vi "Firmware.vi"() -> ()   [LabVIEW 2025]
doc: "VI para instalar el Firmware en las ESP32 \nCon la opcion de subir el firmware en modo Online u Offline"
panel:
  in  "Stop Button":bool
  out "Progreso":u8(slide) scale=0.0..100.0
  out "Compilado":bool
  out "Subido":bool
  in  "Upload Firmware":bool
  out "Lista de COMs":string[](array[string])
  out "error out":errorcluster
  in  "Selector":string(combo)
  # "Instalador de Firmware de Labview ESP32"
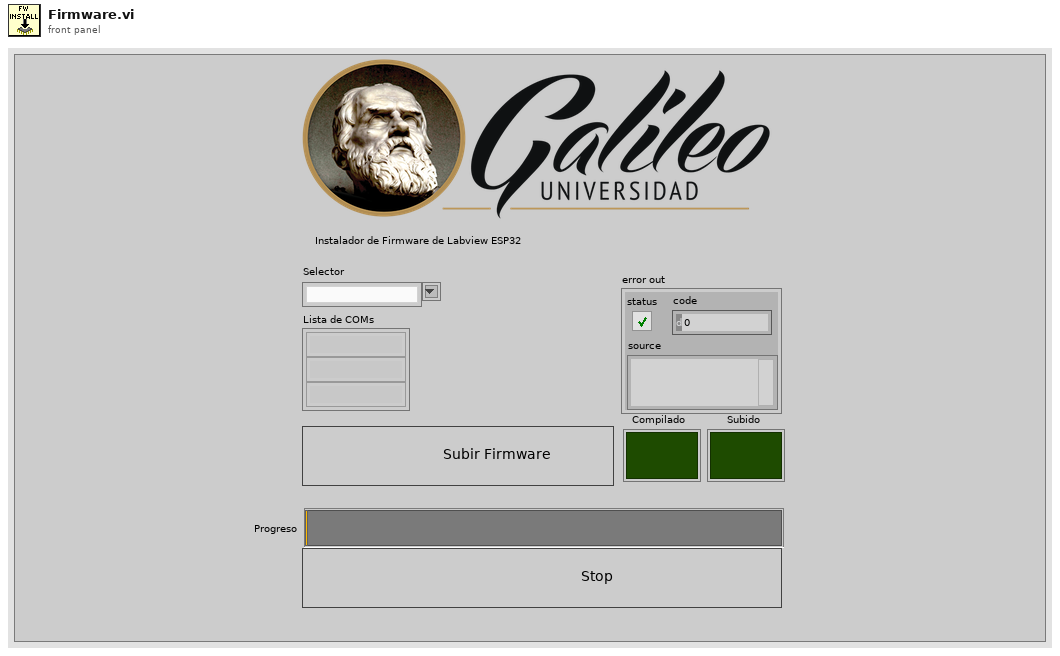
[diagram p1: front panel]
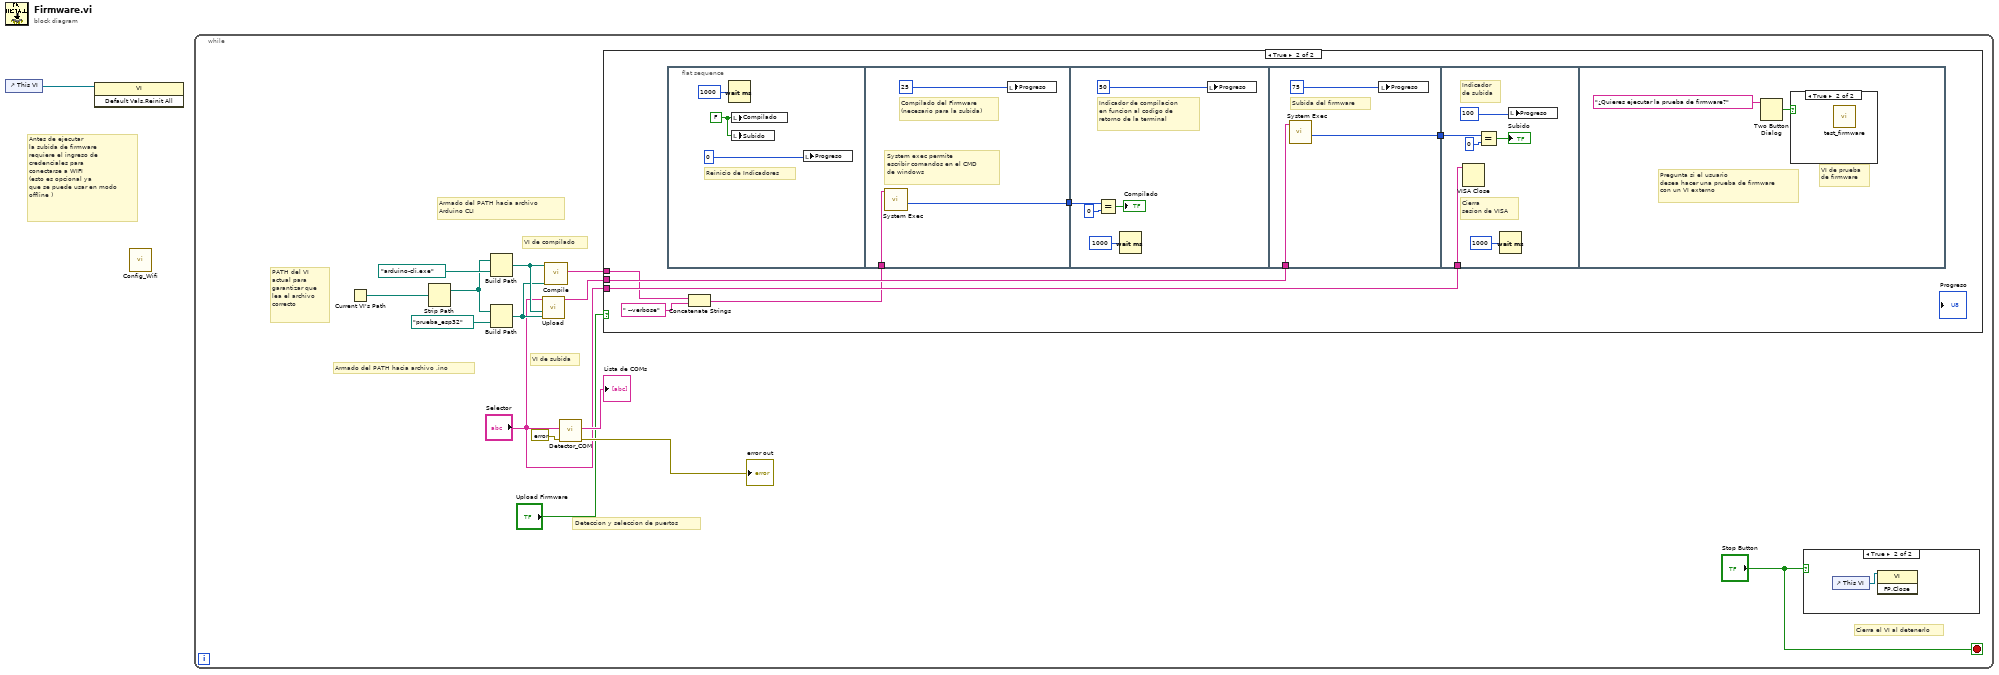
[diagram p0: block diagram]
diagram:
  # "Antes de ejecutar\nla subida de firmware\nrequiere el ingreso de\ncredenciales para \nconectarse a WIFI\n(esto es opcional ya \nque se puede usar en modo \noffline )"
  n1 = control-ref of="This VI"() -> (w1:refnum<vi>)
  n2 = invoke class="VI" method="Default Vals.Reinit All"(reference=w1) -> ()  [unwired: 2 in, 3 out]
  n3 = call "Config_Wifi.vi"() -> ()  [unwired: 12 in]
  n4 = while {
    stop <- "Stop Button" stop-if-true
    # "Cierra el VI al detenerlo"
    # "VI de subida"
    # "VI de compilado"
    # "PATH del VI\nactual para\ngarantizar que \nlea el archivo \ncorrecto"
    # "Armado del PATH hacia archivo \nArduino CLI"
    # "Armado del PATH hacia archivo .ino"
    # "Deteccion y seleccion de puertos"
    n5 = Current VI's Path() -> (path=w13:path)
    n6 = Strip Path(path=w13) -> (stripped path=w10:path)  [unwired: 1 out]
    n7 = Build Path(base path=w10, name or relative path=path "arduino-cli.exe") -> (appended path=w9:path)
    n8 = Build Path(base path=w10, name or relative path=path "prueba_esp32") -> (appended path=w8:path)
    n9 = call "Upload.vi"("INO"=w8, "CLI"=w9, "Selector"="Selector") -> ("Comando_Upload"=w4:string)  [unwired: 8 in]
    n10 = call "Compile.vi"("INO"=w8, "CLI"=w9) -> ("Comando_Compile"=w5:string)  [unwired: 9 in]
    n11 = call "Detector_COM.vi"("error in (no error)"=errorcluster {"status"=FALSE, "code"=0, "source"=""}, "Selector"="Selector") -> ("error out"=→"error out":errorcluster, "find list"=→"Lista de COMs":string[])  [unwired: 8 in]
    n12 = case shown="True" "Upload Firmware" {
      tunnel: w5 -> [_ w19]
      tunnel: w4 -> [_ w21]
      tunnel: "Selector" -> [_ w20]
      frame False {
      }
      frame True {
        n13 = flat-sequence {
          tunnel: [w29] -> w22
          tunnel: w18 -> [w28]
          tunnel: w22 -> [w32]
          tunnel: w21 -> [w37]
          tunnel: [w36] -> w23
          tunnel: w23 -> [w43]
          tunnel: w20 -> [w38]
          frame #0 {
            w26 = FALSE
            # "Reinicio de Indicadores"
            n14 = Wait (ms)(milliseconds to wait=u32 1000) -> ()  [unwired: 1 out]
            n15 = local write "Compilado"(w26) -> ()
            n16 = local write "Subido"(w26) -> ()
            n17 = local write "Progreso"(u8 0 ("Progreso")) -> ()
          }
          frame #1 {
            # "System exec permite\nescribir comandos en el CMD\nde windows"
            # "Compilado del Firmware\n(necesario para la subida)"
            n18 = call <vilib>:"System Exec.vi"("command line"=w28) -> ("return code"=w29:i32)  [unwired: 7 in, 3 out]
            n19 = local write "Progreso"(u8 25 ("Progreso")) -> ()
          }
          frame #2 {
            # "Indicador de compilacion \nen funcion al codigo de\nretorno de la terminal"
            n20 = Equal?(x=w32, y=0) -> (x = y?=→"Compilado":bool)
            n21 = Wait (ms)(milliseconds to wait=u32 1000) -> ()  [unwired: 1 out]
            n22 = local write "Progreso"(u8 50 ("Progreso")) -> ()
          }
          frame #3 {
            # "Subida del firmware"
            n23 = call <vilib>:"System Exec.vi"("command line"=w37) -> ("return code"=w36:i32)  [unwired: 7 in, 3 out]
            n24 = local write "Progreso"(u8 75 ("Progreso")) -> ()
          }
          frame #4 {
            # "Cierra \nsesion de VISA"
            # "Indicador\nde subida"
            n25 = VISA Close(VISA resource name=w38) -> ()  [unwired: 1 in, 1 out]
            n26 = Equal?(x=w43, y=0) -> (x = y?=→"Subido":bool)
            n27 = Wait (ms)(milliseconds to wait=u32 1000) -> ()  [unwired: 1 out]
            n28 = local write "Progreso"(u8 100 ("Progreso")) -> ()
          }
          frame #5 {
            # "VI de prueba\nde firmware"
            # "Pregunta si el usuario\ndesea hacer una prueba de firmware\ncon un VI externo"
            n29 = Two Button Dialog(message="¿Quieres ejecutar la prueba de firmware?") -> (T button?=w45:bool)  [unwired: 2 in]
            n30 = case shown="True" w45 {
              frame False {
              }
              frame True {
                n31 = call "test_firmware.vi"() -> ()  [unwired: 12 in]
              }
            }
          }
        }
        n32 = Concatenate Strings(w19, " --verbose") -> (w18:string)
      }
    }
    n33 = case shown="True" "Stop Button" {
      frame False {
      }
      frame True {
        n34 = control-ref of="This VI"() -> (w16:refnum<vi>)
        n35 = invoke class="VI" method="FP.Close"(reference=w16) -> ()  [unwired: 2 in, 3 out]
      }
    }
  }
